vi "delete_subtable_item.vi"(7 "subtables":string[](array[string]), 8 "error in (no error)":errorcluster, 10 "subkeys":string[](array[string]), 11 "toml in":refnum<class "toml.lvclass">) -> (0 "error out":errorcluster, 2 "deleted?":bool, 3 "toml out":refnum<class "toml.lvclass">)   [LabVIEW 2020, in "toml.lvclass"]
uses:
  toml.lvclass
  toml.lvclass/toml.ctl
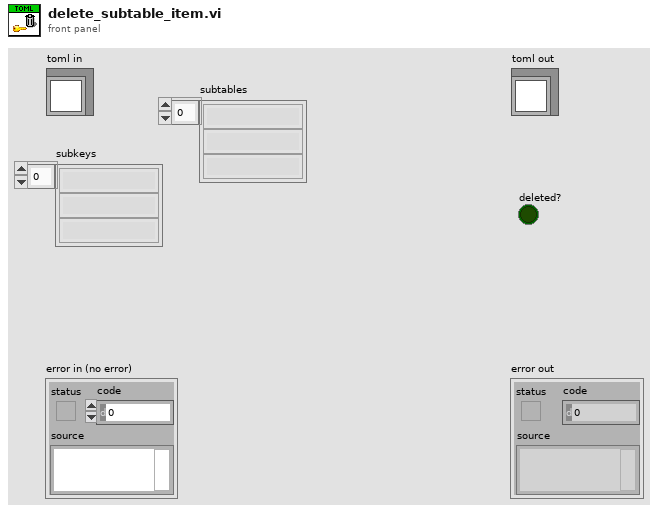
[diagram p1: front panel]
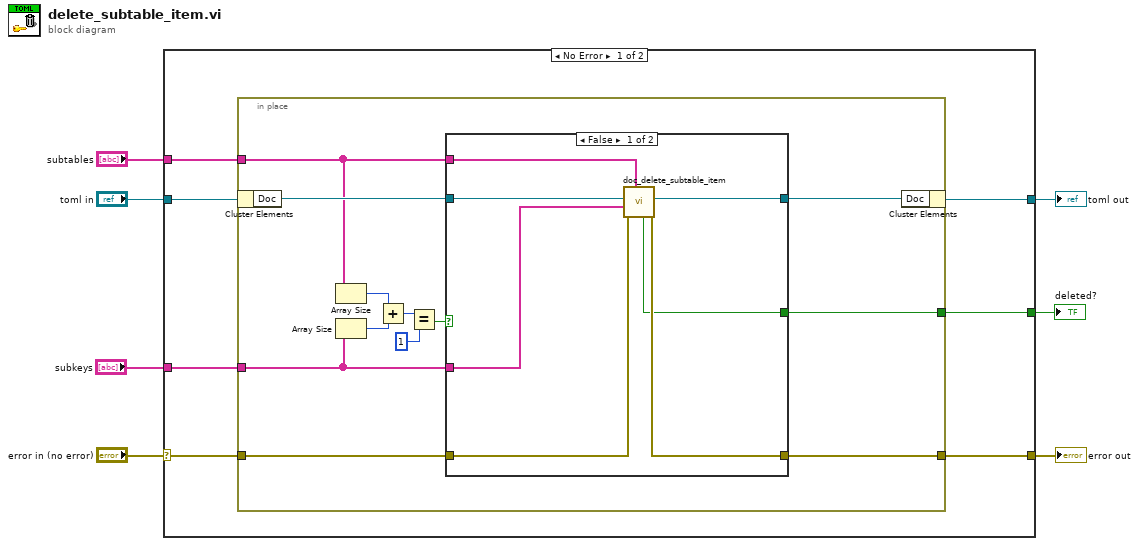
[diagram p0: block diagram]
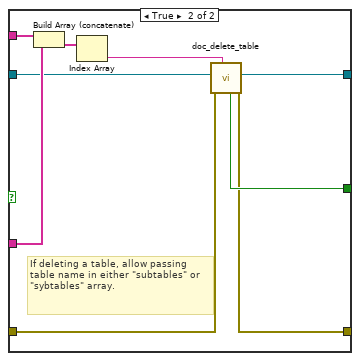
[diagram p2: hidden frame]
diagram:
  n1 = case shown="No Error" "error in (no error)" {
    selector: "error in (no error)" -> [w9 w44]
    tunnel: [w10 w44] -> w6
    tunnel: [w13 w43] -> w4
    tunnel: "toml in" -> [w14 w43]
    tunnel: "subtables" -> [w12 _]
    tunnel: "subkeys" -> [w11 _]
    tunnel: [w8 _] -> w1
    frame No Error {
      n2 = in-place {
        in-place-border: w12 -> [w21]
        in-place-border: w11 -> [w20]
        in-place-border: [w25] -> w10
        in-place-border: w9 -> [w26]
        in-place-border: [w22] -> w8
        n3 = in-place-cluster #1(w14) -> ("Doc"=w24:refnum<class "Doc.lvclass">)
        n4 = Array Size(array=w21) -> (size(s)=w19:i32)
        n5 = Array Size(array=w20) -> (size(s)=w18:i32)
        n6 = Add(x=w19, y=w18) -> (x+y=w17:i32)
        n7 = Equal?(x=w17, y=1) -> (x = y?=w15:bool)
        n8 = case shown="False" w15 {
          tunnel: w26 -> [w33 w36]
          tunnel: [w32 w34] -> w25
          tunnel: w24 -> [w31 w40]
          tunnel: [w30 w39] -> w23
          tunnel: [w29 w35] -> w22
          tunnel: w21 -> [w28 w42]
          tunnel: w20 -> [w27 w41]
          frame False {
            n9 = call "doc_delete_subtable_item.vi"("subtables"=w28, "error in (no error)"=w33, "subkeys"=w27, "Doc in"=w31) -> ("error out"=w32:errorcluster, "Doc out"=w30:refnum<class "Doc.lvclass">, "found?"=w29:bool)  [unwired: 5 in]
          }
          frame True {
            # "If deleting a table, allow passing table name in either \"subtables\" or \"sybtables\" array."
            n10 = Build Array (concatenate)(w42, w41) -> (w38:string[])
            n11 = Index Array(array=w38) -> (element=w37:string)  [unwired: 1 in]
            n12 = call "doc_delete_table.vi"("table"=w37, "error in (no error)"=w36, "Doc in"=w40) -> ("error out"=w34:errorcluster, "Doc out"=w39:refnum<class "Doc.lvclass">, "deleted?"=w35:bool)  [unwired: 6 in]
          }
        }
        n13 = in-place-cluster #1("Doc"=w23) -> (w13:refnum<class "toml.lvclass">)
      }
    }
    frame Error {
    }
  }
  "error out" <- w6
  "toml out" <- w4
  "deleted?" <- w1
